vi "Get Registered Path.vi"(10 "error in (no error)":errorcluster, 11 "Key":variant) -> (2 "error out":errorcluster, 3 "Registered Path":path, 5 "Key Not Found?":bool)   [LabVIEW 2021, in "Path Utilities.lvlib"]
doc: "Return the Registered Path associated to the given Key.\nIf the Key is not found, the corresponding indicator is set to True and Not A Path is returned.\n\nUse \"Register Path.vi\" to register a Path.\nNo error is returned."
uses:
  Path Utilities.lvlib
  TypeDefs/FGV State - Path Registration.ctl
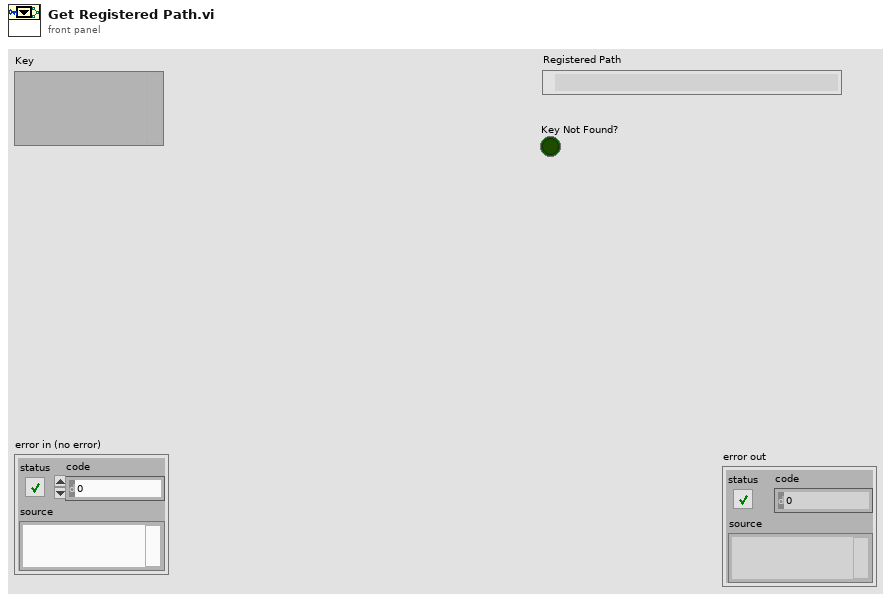
[diagram p1: front panel]
types:
  T1 = typedef "Path Utilities.lvlib/FGV State - Path Registration.ctl" = enum16{"Get Path", "List All Paths", "Register Path", "Unregister Path", "Empty Map"}
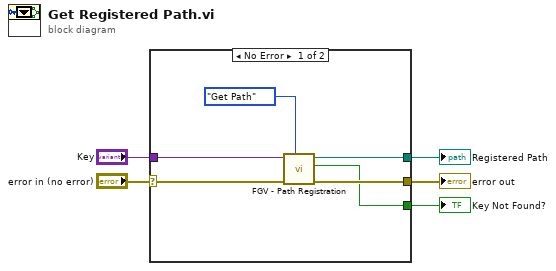
[diagram p0: block diagram]
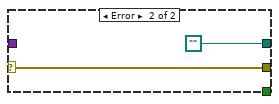
[diagram p2: hidden frame]
diagram:
  n1 = case shown="No Error" "error in (no error)" {
    selector: "error in (no error)" -> [w11 w13]
    tunnel: [w10 w13] -> w4
    tunnel: "Key" -> [w9 _]
    tunnel: [w7 path ""] -> w2
    tunnel: [w6 _] -> w1
    frame No Error {
      n2 = call "FGV - Path Registration.vi"("FGV State"=FGV_State_-_Path_Registration."Get Path", "error in (no error)"=w11, "Key"=w9) -> ("error out"=w10:errorcluster, "Key Not Found?"=w6:bool, "Path Out"=w7:path)  [unwired: 3 in, 3 out]
    }
    frame Error {
    }
  }
  "error out" <- w4
  "Registered Path" <- w2
  "Key Not Found?" <- w1
